vi "Event Log.Destroy.vi"(8 "error in (no error)":errorcluster) -> (0 "error out":errorcluster)   [LabVIEW 2024, in "EQMF.lvlib" / "Event Log.lvlib"]
uses:
  Event Log.lvlib
  Queues/Q.Element.ctl
  Queues/Queue Utils.lvlib
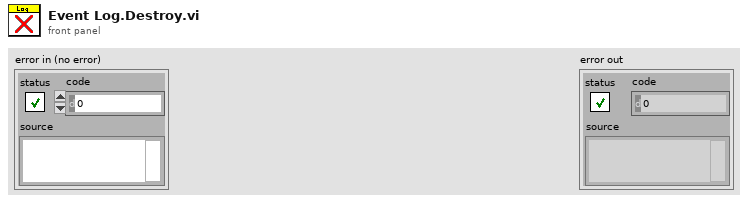
[diagram p1: front panel]
types:
  T1 = typedef "EQMF.lvlib/Queue Utils.lvlib/Q.Element.ctl" = cluster{"Cmd":string, "Sub":string, "Data1":variant, "Data2":variant}
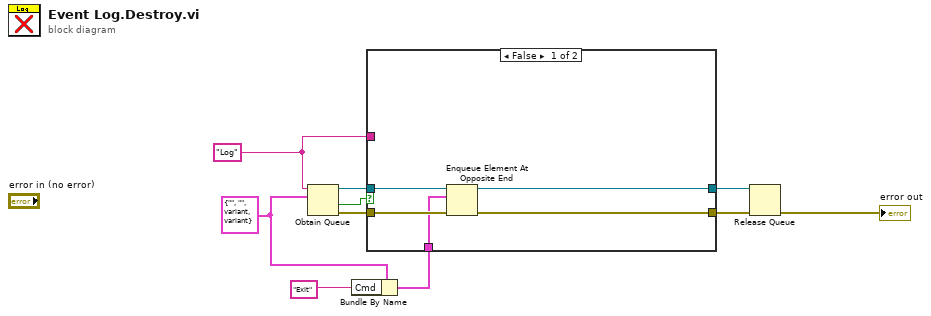
[diagram p0: block diagram]
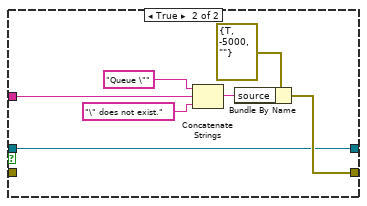
[diagram p2: hidden frame]
diagram:
  w1 = T1 {"Cmd"="", "Sub"="", "Data1"=variant, "Data2"=variant} ("Queue Element")
  w2 = "Log" ("name (unnamed)")
  n1 = Obtain Queue(name (unnamed)=w2, element data type=w1) -> (queue out=w9:refnum<queue>, created new?=w8:bool, error out=w10:errorcluster)  [unwired: 3 in]
  n2 = Bundle By Name(cluster=w1, "Cmd"="Exit") -> (w6:T1)
  n3 = case shown="False" w8 {
    tunnel: w10 -> [w14 _]
    tunnel: w9 -> [w15 w16]
    tunnel: [w11 w18] -> w5
    tunnel: w2 -> [_ w17]
    tunnel: w6 -> [w13 _]
    tunnel: [w12 w16] -> w4
    frame False {
      n4 = Enqueue Element At Opposite End(queue=w15, element=w13, error in (no error)=w14) -> (queue out=w12:refnum<queue>, error out=w11:errorcluster)  [unwired: 1 in, 1 out]
    }
    frame True {
      n5 = Concatenate Strings("Queue \"", w17, "\" does not exist.") -> (w19:string)
      n6 = Bundle By Name(cluster=errorcluster {"status"=TRUE, "code"=-5000, "source"=""} ("error constant"), "source"=w19) -> (w18:errorcluster)
    }
  }
  n7 = Release Queue(queue=w4, error in (no error)=w5) -> (error out=→"error out":errorcluster)  [unwired: 1 in, 2 out]
